vi "gRPC.Server.DiscoverPort.vi"(8 "error in (no error)":errorcluster, 10 "Name":string, 11 "IP Address":string) -> (0 "error out":errorcluster, 3 "Port":i32)   [LabVIEW 2025, in "XNET Bus Monitor Client.lvlib"]
uses:
  XNET Bus Monitor Client.lvlib
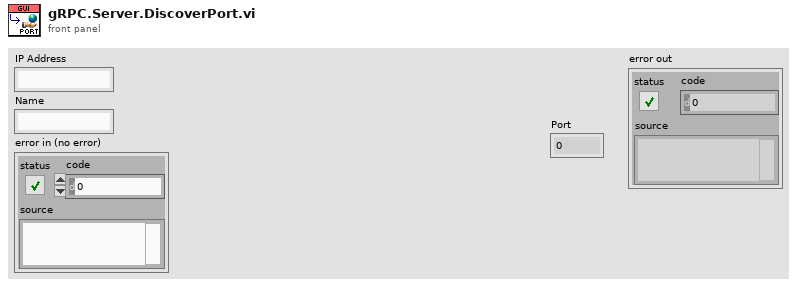
[diagram p1: front panel]
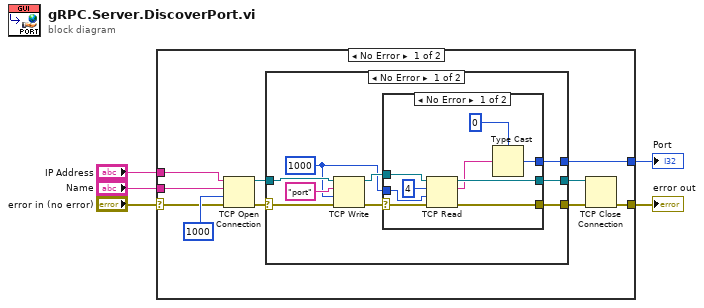
[diagram p0: block diagram]
diagram:
  n1 = case shown="No Error" "error in (no error)" {
    selector: "error in (no error)" -> [w11 w38]
    tunnel: [w10 w38] -> w2
    tunnel: "Name" -> [w8 _]
    tunnel: "IP Address" -> [w7 _]
    tunnel: [w6 _] -> w3
    frame No Error {
      n2 = TCP Open Connection(address=w7, remote port or service name=w8, timeout ms (60000)=1000, error in (no error)=w11) -> (connection ID=w14:refnum<k5>, error out=w9:errorcluster)  [unwired: 1 in]
      n3 = case shown="No Error" w9 {
        selector: w9 -> [w17 w37]
        tunnel: w14 -> [w24 w36]
        tunnel: [w20 w36] -> w13
        tunnel: [w19 w37] -> w12
        tunnel: [w18 _] -> w6
        frame No Error {
          w21 = 1000 ("timeout ms (25000)")
          n4 = TCP Write(connection ID=w24, data in="port", error in (no error)=w17, 9:w21) -> (connection ID out=w22:refnum<k5>, error out=w16:errorcluster)  [unwired: 1 out]
          n5 = case shown="No Error" w16 {
            selector: w16 -> [w25 w35]
            tunnel: w22 -> [w33 w34]
            tunnel: w21 -> [w32 _]
            tunnel: [w30 w34] -> w20
            tunnel: [w29 w35] -> w19
            tunnel: [w26 _] -> w18
            frame No Error {
              n6 = TCP Read(connection ID=w33, bytes to read=4, error in (no error)=w25, 9:w32) -> (connection ID out=w30:refnum<k5>, data out=w28:string, error out=w29:errorcluster)  [unwired: 1 in]
              n7 = Type Cast(type=0, x=w28) -> (*(type *) &x=w26:i32)
            }
            frame Error {
            }
          }
        }
        frame Error {
        }
      }
      n8 = TCP Close Connection(connection ID=w13, error in (no error)=w12) -> (error out=w10:errorcluster)  [unwired: 1 in, 1 out]
    }
    frame Error {
    }
  }
  "error out" <- w2
  "Port" <- w3
